vi "Make Channels Coincident.vi"(8 "interp. method":i32(ring) items=["nearest", "linear", "spline", "cubic Hermite", "Lagrange"], 9 "Cluster 2":T1={"Colour"=0, "Inst type"=enum."Pitot-static tube", "Inst name"="Manometer voltage", "Symbol"="U", "Code name"="", "Extra Info"="U", "Inst Array"=enum."PWA", "Index"=0, "Voltage Index"=0, "Extra Titles"=[], "Extra Values"=[], "Eng Values"=[], "Time (ms)"=[], "TT / Voltage"=[], "U"=0.0, "u^2"=0.0, "u^3"=0.0, "u^4"=0.0, "Skew_u"=0.0, "Kurt_u"=0.0, "Mean % Err"=0.0, "% u'/U"=0.0} {"Skew_u" format="%.2f"; "% u'/U" format="%.2f"; "Mean % Err" format="%.2f"; "Kurt_u" format="%.2f"; "u^4" format="%.2f"; "u^3" format="%.2f"; "U" format="%.2f"; "u^2" format="%.2f"}, 11 "Cluster 1":T1={"Colour"=0, "Inst type"=enum."Pitot-static tube", "Inst name"="Manometer voltage", "Symbol"="U", "Code name"="", "Extra Info"="U", "Inst Array"=enum."PWA", "Index"=0, "Voltage Index"=0, "Extra Titles"=[], "Extra Values"=[], "Eng Values"=[], "Time (ms)"=[], "TT / Voltage"=[], "U"=0.0, "u^2"=0.0, "u^3"=0.0, "u^4"=0.0, "Skew_u"=0.0, "Kurt_u"=0.0, "Mean % Err"=0.0, "% u'/U"=0.0} {"Skew_u" format="%.2f"; "% u'/U" format="%.2f"; "Mean % Err" format="%.2f"; "Kurt_u" format="%.2f"; "u^4" format="%.2f"; "u^3" format="%.2f"; "U" format="%.2f"; "u^2" format="%.2f"}) -> (1 "Coincident Channel 2":T1={"Colour"=0, "Inst type"=enum."Pitot-static tube", "Inst name"="Manometer voltage", "Symbol"="U", "Code name"="", "Extra Info"="U", "Inst Array"=enum."PWA", "Index"=0, "Voltage Index"=0, "Extra Titles"=[], "Extra Values"=[], "Eng Values"=[], "Time (ms)"=[], "TT / Voltage"=[], "U"=0.0, "u^2"=0.0, "u^3"=0.0, "u^4"=0.0, "Skew_u"=0.0, "Kurt_u"=0.0, "Mean % Err"=0.0, "% u'/U"=0.0} {"Skew_u" format="%.2f"; "% u'/U" format="%.2f"; "Mean % Err" format="%.2f"; "Kurt_u" format="%.2f"; "u^4" format="%.2f"; "u^3" format="%.2f"; "U" format="%.2f"; "u^2" format="%.2f"}, 3 "Coincident Channel 1":T1={"Colour"=0, "Inst type"=enum."Pitot-static tube", "Inst name"="Manometer voltage", "Symbol"="U", "Code name"="", "Extra Info"="U", "Inst Array"=enum."PWA", "Index"=0, "Voltage Index"=0, "Extra Titles"=[], "Extra Values"=[], "Eng Values"=[], "Time (ms)"=[], "TT / Voltage"=[], "U"=0.0, "u^2"=0.0, "u^3"=0.0, "u^4"=0.0, "Skew_u"=0.0, "Kurt_u"=0.0, "Mean % Err"=0.0, "% u'/U"=0.0} {"Skew_u" format="%.2f"; "% u'/U" format="%.2f"; "Mean % Err" format="%.2f"; "Kurt_u" format="%.2f"; "u^4" format="%.2f"; "u^3" format="%.2f"; "U" format="%.2f"; "u^2" format="%.2f"})   [LabVIEW 2011]
uses:
  Controls/Analysis_info_cluster.ctl
  Controls/Inst_type.ctl
  Controls/Instrument_Array.ctl
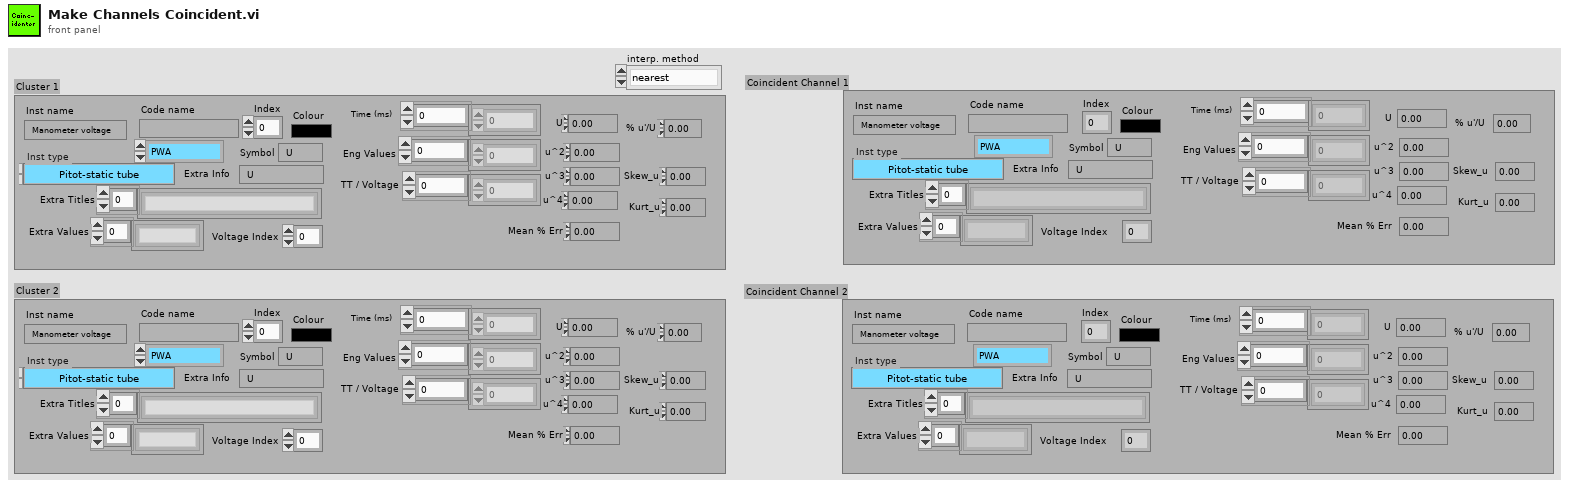
[diagram p1: front panel]
types:
  T1 = typedef "Analysis_info_cluster.ctl" = cluster{"Colour":u32, "Inst type":T2, "Inst name":string, "Symbol":string, "Code name":string, "Extra Info":string, "Inst Array":T3, "Index":i32, "Voltage Index":i32, "Extra Titles":string[], "Extra Values":string[], "Eng Values":dbl[], "Time (ms)":dbl[], "TT / Voltage":dbl[], "U":dbl, "u^2":dbl, "u^3":dbl, "u^4":dbl, "Skew_u":dbl, "Kurt_u":dbl, "Mean % Err":dbl, "% u'/U":dbl}
  T2 = typedef "Inst_type.ctl" = enum16{"Propeller anemometer", "Raw voltage", "Pressure Transducer", "Pitot-static tube", "Preston tube", "Hot wire", "Cross wire 1", "Cross wire 2", "Generic Linear", "Generic Polynomial", "Generic BackPoly", "Fast FID", "Thermocouple", "Cold wire", "Pulsed Wire", "LDA Vel", "LDA Tran time", "LDA Arr time"}
  T3 = typedef "Instrument_Array.ctl" = enum16{"PWA", "LDA", "Analogue"}
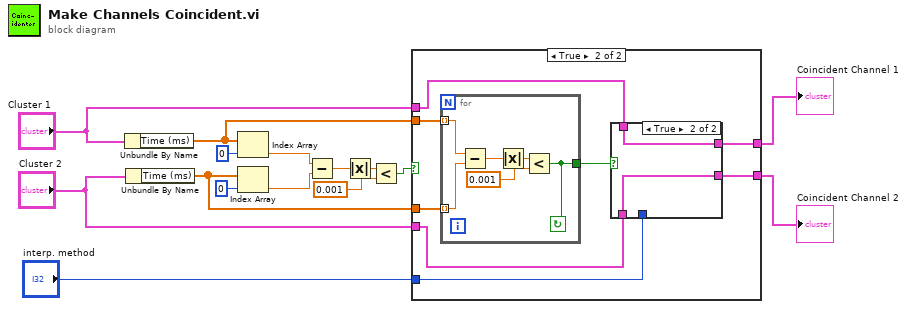
[diagram p0: block diagram]
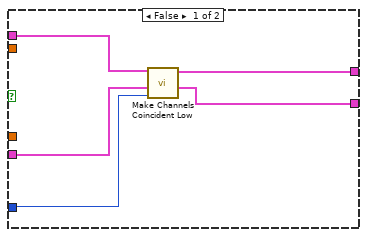
[diagram p2: hidden frame]
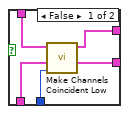
[diagram p3: hidden frame]
diagram:
  n1 = Unbundle By Name("Cluster 1") -> ("Time (ms)"=w11:dbl[])
  n2 = Unbundle By Name("Cluster 2") -> ("Time (ms)"=w10:dbl[])
  n3 = Index Array(array=w11, index=0) -> (element=w13:dbl)
  n4 = Index Array(array=w10, index=0) -> (element=w12:dbl)
  n5 = Subtract(x=w13, y=w12) -> (x-y=w4:dbl)
  n6 = Absolute Value(x=w4) -> (abs(x)=w3:dbl)
  n7 = Less?(x=w3, y=0.001) -> (x < y?=w1:bool)
  n8 = case shown="True" w1 {
    tunnel: w11 -> [_ w28]
    tunnel: w10 -> [_ w27]
    tunnel: "Cluster 1" -> [w20 w24]
    tunnel: "Cluster 2" -> [w19 w25]
    tunnel: [w18 w23] -> w7
    tunnel: [w17 w22] -> w6
    tunnel: "interp. method" -> [w16 w21]
    frame False {
      n9 = call "Make Channels Coincident Low.vi"("interp. method"=w16, "Cluster 2"=w19, "Cluster 1"=w20) -> ("Coincident Channel 2"=w17:T1, "Coincident Channel 1"=w18:T1)  [unwired: 7 in]
    }
    frame True {
      n10 = for {
        tunnel: w28 -> [w38] mode=indexing
        tunnel: w27 -> [w37] mode=indexing
        tunnel: [w36] -> w26
        stop <- w36 continue-if-true
        n11 = Subtract(x=w38, y=w37) -> (x-y=w41:dbl)
        n12 = Absolute Value(x=w41) -> (abs(x)=w40:dbl)
        n13 = Less?(x=w40, y=0.001) -> (x < y?=w36:bool)
      }
      n14 = case shown="True" w26 {
        tunnel: w24 -> [w32 w35]
        tunnel: w25 -> [w33 w34]
        tunnel: [w31 w35] -> w23
        tunnel: [w30 w34] -> w22
        tunnel: w21 -> [w29 _]
        frame False {
          n15 = call "Make Channels Coincident Low.vi"("interp. method"=w29, "Cluster 2"=w33, "Cluster 1"=w32) -> ("Coincident Channel 2"=w30:T1, "Coincident Channel 1"=w31:T1)  [unwired: 7 in]
        }
        frame True {
        }
      }
    }
  }
  "Coincident Channel 1" <- w7
  "Coincident Channel 2" <- w6
